vi "Actor Create.vi"(9 "Nested Alias":string, 10 "Nested Actor":refnum<class "Actor.lvclass">, 11 "Self Actor in":refnum<class "Self Actor.lvclass">) -> (0 "error out":errorcluster, 3 "Self Actor out":refnum<class "Self Actor.lvclass">)   [LabVIEW 2021, in "jettl.lvlib" / "Self Actor.lvclass"]
uses:
  Self Actor.lvclass
  C:/git/jettl/src/LVCAM/LVCAM/Actor/Actor.lvclass
  Actor/Actor.lvclass
  Msging Self Actor State/Msging Self Actor State.lvclass
  C:/git/jettl/src/LVCAM/LVCAM/Self Actor State/Self Actor State.lvclass
  Self Actor.lvclass/Self Actor.ctl
  Actor/Actor Loop.vi
  jettl.lvlib
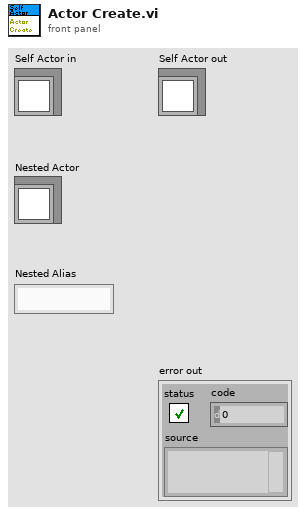
[diagram p1: front panel]
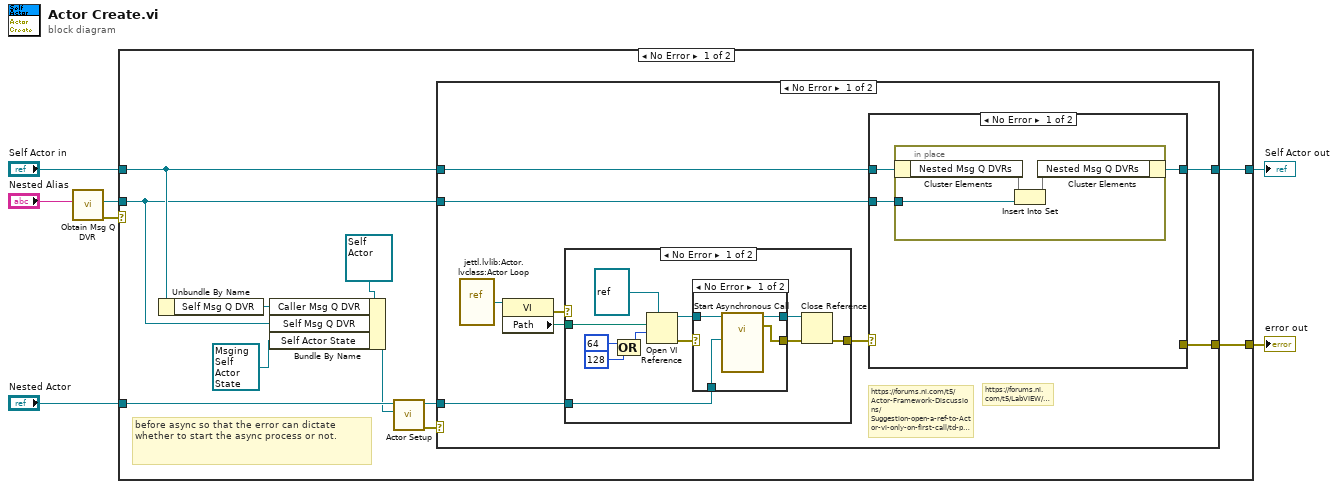
[diagram p0: block diagram]
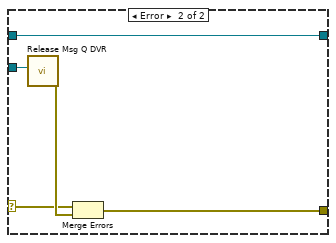
[diagram p4: hidden frame]
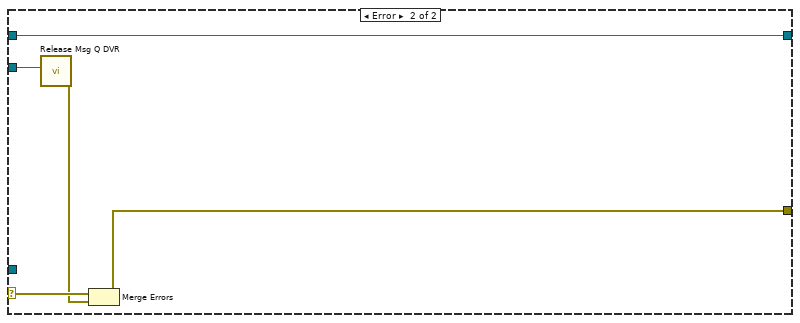
[diagram p5: hidden frame]
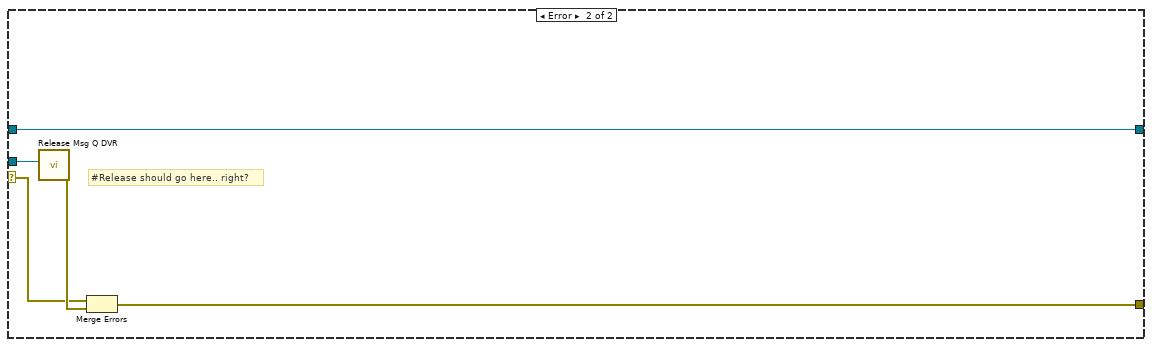
[diagram p6: hidden frame]
diagram:
  n1 = call "Obtain Msg Q DVR.vi"("Msg Q DVR Alias"="Nested Alias") -> ("error out"=w1:errorcluster, "Msg Q DVR"=w3:refnum<data-value>)  [unwired: 9 in]
  n2 = case shown="No Error" w1 {
    selector: w1 -> [_ w62]
    tunnel: [w18 w66] -> w7
    tunnel: [w16 w64] -> w4
    tunnel: "Nested Actor" -> [w14 _]
    tunnel: w3 -> [w11 w65]
    tunnel: "Self Actor in" -> [w13 w66]
    frame No Error {
      # "before async so that the error can dictate whether to start the async process or not."
      n3 = Unbundle By Name(w13) -> ("Self Msg Q DVR"=w12:refnum<data-value>)
      n4 = Bundle By Name(cluster=refnum<class "Self Actor.lvclass"> refnum ("Self Actor in"), "Caller Msg Q DVR"=w12, "Self Msg Q DVR"=w11, "Self Actor State"=refnum<class "Msging Self Actor State.lvclass"> refnum ("LVCAM.lvlib:Msging Self Actor State.lvclass")) -> (w10:refnum<class "Self Actor.lvclass">)
      n5 = call-dynamic "Actor Setup.vi"("Actor"=w10, "Actor in"=w14) -> ("error out"=w9:errorcluster, "Actor out"=w17:refnum<class "Actor.lvclass">)  [unwired: 8 in]
      n6 = case shown="No Error" w9 {
        selector: w9 -> [_ w61]
        tunnel: [w27 w59] -> w18
        tunnel: w17 -> [w26 _]
        tunnel: [w25 w58] -> w16
        tunnel: w13 -> [w23 w59]
        tunnel: w11 -> [w22 w60]
        frame No Error {
          # "https://forums.ni.com/t5/LabVIEW/Static-VI-Reference/m-p/3334014#M978333"
          # "https://forums.ni.com/t5/Actor-Framework-Discussions/Suggestion-open-a-ref-to-Actor-vi-only-on-first-call/td-p/3451643/page/4"
          n7 = vi-ref "jettl.lvlib:Actor.lvclass:Actor Loop.vi"() -> (w20:refnum<vi>)
          n8 = property class="VI"(reference=w20) -> (error out=w21:errorcluster, "Path"=w19:path)  [unwired: 1 in, 1 out]
          n9 = case shown="No Error" w21 {
            selector: w21 -> [_ w45]
            tunnel: [w36 w45] -> w24
            tunnel: w19 -> [w32 _]
            tunnel: w26 -> [w28 _]
            frame No Error {
              n10 = Compound Arithmetic op=OR(64 ("options: Multiple Clones,\n  Fire & Forget"), 128 ("options: Multiple Clones,\n  Fire & Forget")) -> (w34:i32)
              n11 = Open VI Reference(type specifier VI Refnum (for type only)=refnum<vi> refnum, vi path=w32, options=w34) -> (vi reference=w30:refnum<vi>, error out=w31:errorcluster)  [unwired: 3 in]
              n12 = case shown="No Error" w31 {
                selector: w31 -> [_ w44]
                tunnel: [w42 w43] -> w38
                tunnel: [w41 w44] -> w37
                tunnel: w30 -> [w40 w43]
                tunnel: w28 -> [w39 _]
                frame No Error {
                  n13 = call-by-ref "Start Asynchronous Call"(reference=w40, "Actor in"=w39) -> (reference out=w42:refnum<vi>, error out=w41:errorcluster)  [unwired: 12 in]
                }
                frame Error {
                }
              }
              n14 = Close Reference(reference=w38, error in (no error)=w37) -> (error out=w36:errorcluster)
            }
            frame Error {
            }
          }
          n15 = case shown="No Error" w24 {
            selector: w24 -> [_ w52]
            tunnel: w23 -> [w48 w56]
            tunnel: [w47 w56] -> w27
            tunnel: w22 -> [w46 w55]
            tunnel: [_ w54] -> w25
            frame No Error {
              n16 = in-place {
                in-place-border: w46 -> [w49]
                n17 = in-place-cluster #1(w48) -> ("Nested Msg Q DVRs"=w51:set{refnum<data-value>})
                n18 = Insert Into Set(10:w49, 11:w51) -> (3:w50:set{refnum<data-value>})  [unwired: 1 out]
                n19 = in-place-cluster #1("Nested Msg Q DVRs"=w50) -> (w47:refnum<class "Self Actor.lvclass">)
              }
            }
            frame Error {
              n20 = call "Release Msg Q DVR.vi"("Msg Q DVR"=w55) -> ("error out"=w53:errorcluster)  [unwired: 10 in]
              n21 = Merge Errors(w52, w53) -> (w54:errorcluster)
            }
          }
        }
        frame Error {
          n22 = call "Release Msg Q DVR.vi"("Msg Q DVR"=w60) -> ("error out"=w57:errorcluster)  [unwired: 10 in]
          n23 = Merge Errors(w61, w57) -> (w58:errorcluster)
        }
      }
    }
    frame Error {
      # "#Release should go here.. right?"
      n24 = call "Release Msg Q DVR.vi"("Msg Q DVR"=w65) -> ("error out"=w63:errorcluster)  [unwired: 10 in]
      n25 = Merge Errors(w62, w63) -> (w64:errorcluster)
    }
  }
  "error out" <- w4
  "Self Actor out" <- w7
